vi "RSD_up.vi"(2 "S":bool, 3 "C":bool, 4 "D":bool, 5 "R":bool) -> (0 "!Q":bool, 1 "Q":bool)   [LabVIEW 2013]
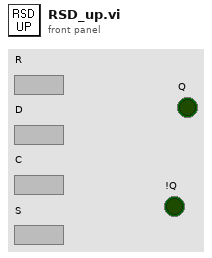
[diagram p1: front panel]
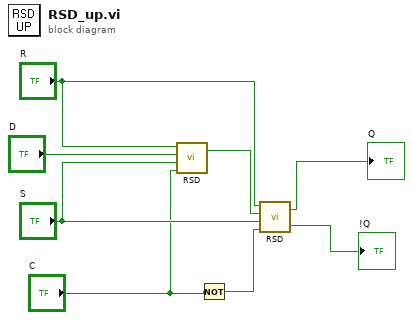
[diagram p0: block diagram]
diagram:
  n1 = call "RSD.vi"("C"="C", "S"="S", "D"="D", "R"="R") -> ("Q"=w5:bool)  [unwired: 1 out]
  n2 = Not(x="C") -> (.not. x?=w2:bool)
  n3 = call "RSD.vi"("C"=w2, "S"="S", "D"=w5, "R"="R") -> ("!Q"=→"!Q":bool, "Q"=→"Q":bool)
